vi "Analyze Target.vi"(8 "Goal Width":dbl, 9 "Center Right":dbl, 10 "Center Left":dbl, 11 "Relevant Data":T1(array[cluster])) -> (3 "What to do":string)   [LabVIEW 2015]
panel:
  in  "Goal Area":dbl
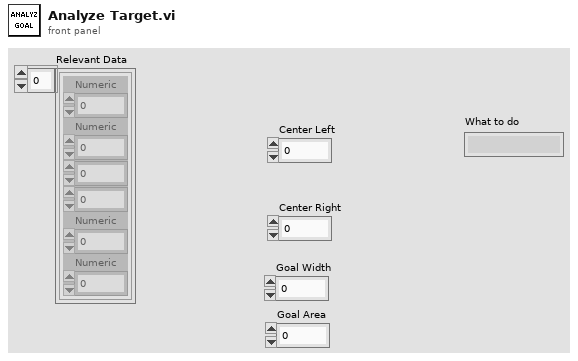
[diagram p1: front panel]
types:
  T1 = cluster{"Numeric":dbl, "Numeric":dbl, dbl, dbl, "Numeric":dbl, "Numeric":dbl}[]
  T2 = cluster{"Numeric":dbl, "Numeric":dbl, dbl, dbl, "Numeric":dbl, "Numeric":dbl}
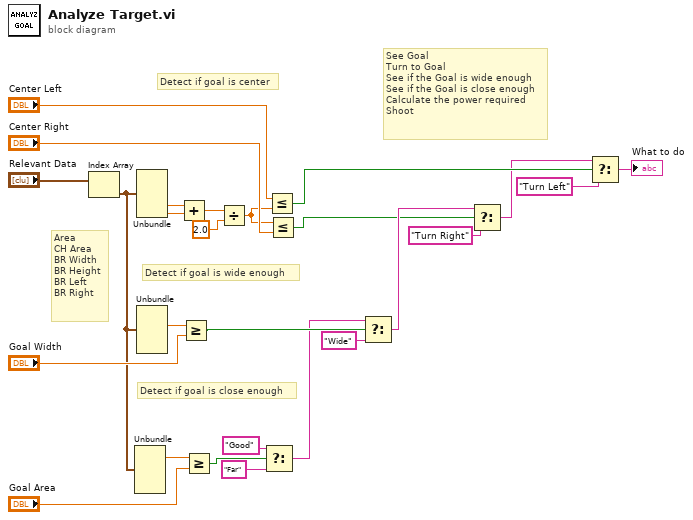
[diagram p0: block diagram]
diagram:
  # "See Goal\nTurn to Goal\nSee if the Goal is wide enough\nSee if the Goal is close enough\nCalculate the power required\nShoot"
  # "Detect if goal is close enough"
  # "Detect if goal is wide enough"
  # "Detect if goal is center"
  # "Area\nCH Area\nBR Width\nBR Height\nBR Left\nBR Right"
  n1 = Index Array(array="Relevant Data") -> (element=w15:T2)  [unwired: 1 in]
  n2 = Unbundle(w15) -> ("Numeric"=w14:dbl)  [unwired: 5 out]
  n3 = Unbundle(w15) -> ("Numeric"=w21:dbl, "Numeric"=w20:dbl)  [unwired: 4 out]
  n4 = Unbundle(w15) -> (w16:dbl)  [unwired: 5 out]
  n5 = Add(x=w21, y=w20) -> (x+y=w19:dbl)
  n6 = Greater Or Equal?(x=w16, y="Goal Width") -> (x >= y?=w9:bool)
  n7 = Greater Or Equal?(x=w14, y="Goal Area") -> (x >= y?=w13:bool)
  n8 = Divide(x=w19, y=2.0) -> (x/y=w17:dbl)
  n9 = Select(t="Good", s=w13, f="Far") -> (s? t:f=w8:string)
  n10 = Less Or Equal?(x="Center Left", y=w17) -> (x <= y?=w3:bool)
  n11 = Less Or Equal?(x=w17, y="Center Right") -> (x <= y?=w4:bool)
  n12 = Select(t=w8, s=w9, f="Wide") -> (s? t:f=w6:string)
  n13 = Select(t=w6, s=w4, f="Turn Right") -> (s? t:f=w2:string)
  n14 = Select(t=w2, s=w3, f="Turn Left") -> (s? t:f=→"What to do":string)
